vi "Close.vi"(8 "error in":errorcluster, 11 "Temperature Gradient in":refnum<class "Temperature Gradient.lvclass">) -> (0 "error out":errorcluster, 3 "Temperature Gradient out":refnum<class "Temperature Gradient.lvclass">)   [LabVIEW 2023, in "Temperature Gradient.lvclass"]
uses:
  Temperature Gradient.lvclass
  Temperature Gradient.lvclass/Temperature Gradient.ctl
  Parents/Gradient/Gradient.lvclass
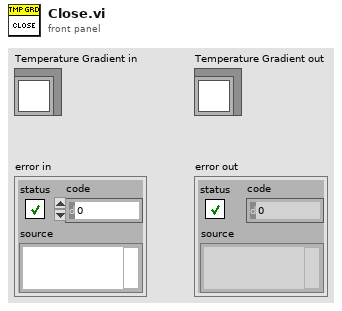
[diagram p1: front panel]
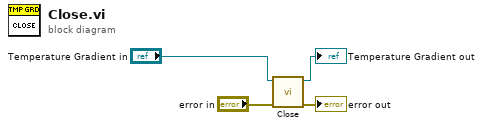
[diagram p0: block diagram]
diagram:
  n1 = call-parent "Close.vi"("error in"="error in", "Gradient in"="Temperature Gradient in") -> ("error out"=→"error out":errorcluster, "Gradient out"=→"Temperature Gradient out":refnum<class "Temperature Gradient.lvclass">)  [unwired: 8 in]
